vi "ABR3-Read Data.vi"(0 "Path":path, 11 "error in (no error)":errorcluster) -> (4 "Header":T3, 6 "Neural":dbl[][](array[numeric]), 8 "CM":dbl[][](array[numeric]), 10 "I-O":dbl[][](array[numeric]), 14 "Analysis":T1, 15 "error out":errorcluster)   [LabVIEW 2020]
uses:
  TypeDefs/ABR3-Analysis State.ctl
  Threshold Estimation VIs/ABR3-Threshold Estimation Result.ctl
  epl-vi-lib/Utility VIs/Array Manipulation VIs/Irregular Array Subset (DBL).vi
  epl-vi-lib/Utility VIs/Array Manipulation VIs/Array-Dimensions (2D).vi
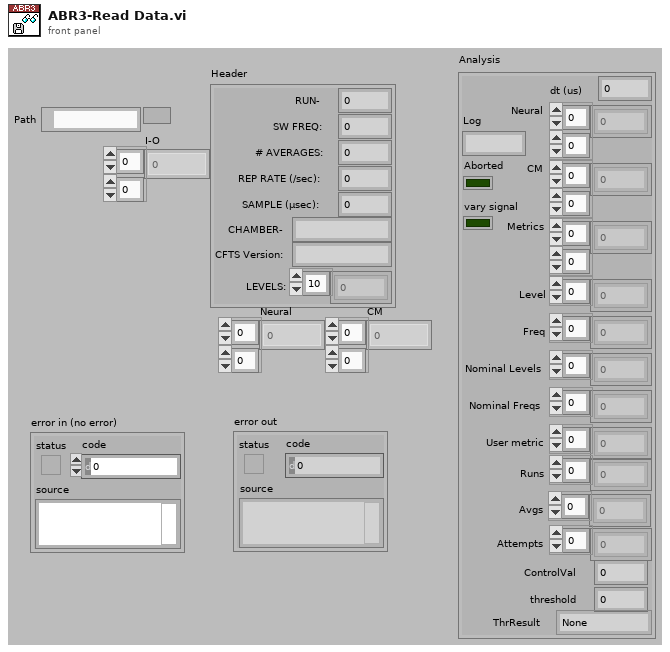
[diagram p1: front panel]
types:
  T1 = typedef "ABR3-Analysis State.ctl" = cluster{"dt (us)":dbl, "Neural":dbl[][], "CM":dbl[][], "Metrics":dbl[][], "Level":dbl[], "Freq":dbl[], "Nominal Levels":dbl[], "Nominal Freqs":dbl[], "User metric":dbl[], "Runs":i32[], "Avgs":i32[], "Attempts":i32[], "Log":string, "Aborted":bool, "ControlVal":dbl, "threshold":dbl, "vary signal":bool, "ThrResult":T2}
  T2 = typedef "ABR3-Threshold Estimation Result.ctl" = enum16{"None", "Power", "Sigmoid", "Power (noisy)", "Suprathreshold", "Invalid"}
  T3 = cluster{"RUN-":i32, "SW FREQ:":dbl, "# AVERAGES:":i32, "REP RATE (/sec):":dbl, "SAMPLE (µsec):":dbl, "CHAMBER-":string, "CFTS Version: ":string, "LEVELS:":dbl[]}
  T4 = typedef "ABR-Data Header.ctl" = cluster{"RUN-":i32, "SW FREQ:":dbl, "# AVERAGES:":i32, "REP RATE (/sec):":dbl, "SAMPLE (µsec):":dbl, "CHAMBER-":string, "CFTS Version: ":string, "LEVELS:":dbl[], "Date":timestamp, "Threshold:":dbl}
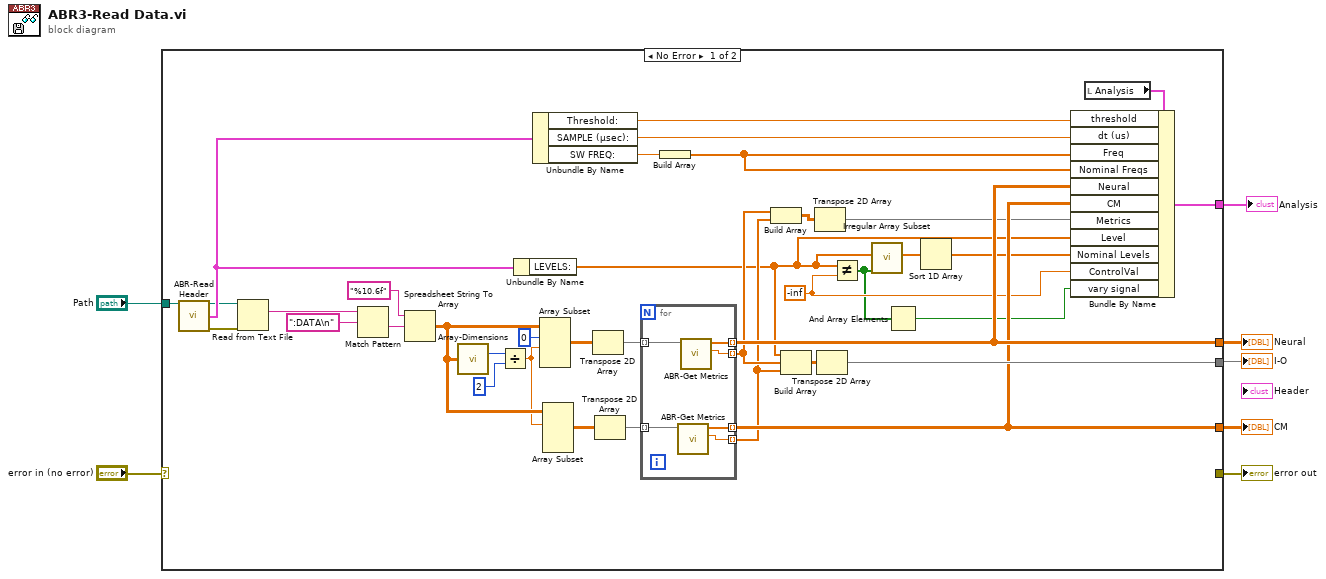
[diagram p0: block diagram]
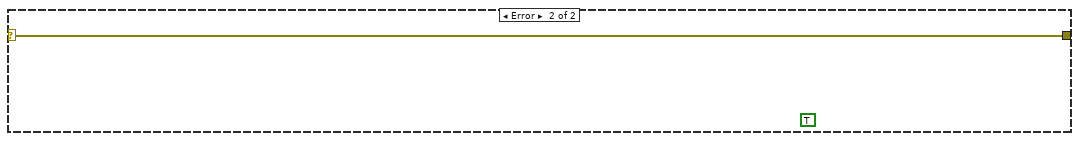
[diagram p2: hidden frame]
diagram:
  n1 = case shown="No Error" "error in (no error)" {
    selector: "error in (no error)" -> [_ w51]
    tunnel: [_ w51] -> w6
    tunnel: "Path" -> [w10 _]
    tunnel: [w41 _] -> w4
    tunnel: [w40 _] -> w3
    tunnel: [w43 _] -> w2
    tunnel: [w42 _] -> w1
    frame No Error {
      w18 = -inf
      n2 = call "ABR-Read Header.vi"("Path"=w10) -> ("Path (thru)"=w11:path, "Header"=w12:T4, "error out"=w9:errorcluster)  [unwired: 12 in]
      n3 = Read from Text File(file (use dialog)=w11, error in=w9) -> (text=w44:string)  [unwired: 2 in, 3 out]
      n4 = Match Pattern(string=w44, regular expression=":DATA\n" ("search string/char (-)")) -> (after substring=w31:string)  [unwired: 1 in, 3 out]
      n5 = Spreadsheet String To Array(format string="%10.6f" ("spreadsheet string"), spreadsheet string=w31) -> (array=w34:dbl[][])  [unwired: 2 in]
      n6 = call-poly "Array-Dimensions.vi"("2D Array"=w34) -> ("# rows"=w38:i32)  [unwired: 13 in, 1 out]
      n7 = Divide(x=w38, y=2) -> (x/y=w32:dbl)
      n8 = Unbundle By Name(w12) -> ("LEVELS:"=w17:dbl[])
      n9 = Unbundle By Name(w12) -> ("Threshold:"=w8:dbl, "SAMPLE (µsec):"=w25:dbl, "SW FREQ:"=w26:dbl)
      n10 = Array Subset(array=w34, index (row)=0 ("index"), length (row)=w32) -> (w35:dbl[][])  [unwired: 2 in]
      n11 = Array Subset(array=w34, index (row)=w32) -> (w33:dbl[][])  [unwired: 3 in]
      n12 = Transpose 2D Array(2D array=w35) -> (transposed array=w29:dbl[][])
      n13 = Transpose 2D Array(2D array=w33) -> (transposed array=w28:dbl[][])
      n14 = for {
        tunnel: w29 -> [w46] mode=indexing
        tunnel: w28 -> [w45] mode=indexing
        tunnel: [w50] -> w41 mode=indexing
        tunnel: [w49] -> w40 mode=indexing
        tunnel: [w48] -> w20 mode=indexing
        tunnel: [w47] -> w19 mode=indexing
        n15 = call "ABR-Get Metrics.vi"("Data in"=w45) -> ("spread value"=w47:dbl, "Data out"=w49:dbl[])  [unwired: 8 in, 1 out]
        n16 = call "ABR-Get Metrics.vi"("Data in"=w46) -> ("spread value"=w48:dbl, "Data out"=w50:dbl[])  [unwired: 8 in, 1 out]
      }
      n17 = Build Array(w26) -> (w24:dbl[])
      n18 = Build Array(w20, w19) -> (w22:dbl[][])
      n19 = Build Array(w17, w20, w19) -> (w27:dbl[][])
      n20 = Transpose 2D Array(2D array=w22) -> (transposed array=w21:dbl[][])
      n21 = Transpose 2D Array(2D array=w27) -> (transposed array=w43:dbl[][])
      n22 = Not Equal?(x=w17, y=w18) -> (x != y?=w14:bool[])
      n23 = call-poly "Irregular Array Subset.vi"("Mask"=w14, "Array"=w17) -> ("Array Subset"=w16:dbl[])  [unwired: 8 in, 1 out]
      n24 = And Array Elements(Boolean array=w14) -> (logical AND=w13:bool)
      n25 = Sort 1D Array(array=w16) -> (sorted array=w15:dbl[])
      n26 = local read "Analysis"() -> (w23:T1)
      n27 = Bundle By Name(cluster=w23, "threshold"=w8, "dt (us)"=w25, "Freq"=w24, "Nominal Freqs"=w24, "Neural"=w41, "CM"=w40, "Metrics"=w21, "Level"=w17, "Nominal Levels"=w15, "ControlVal"=w18, "vary signal"=w13) -> (w42:T1)
    }
    frame Error {
      (unwired) TRUE ("cancelled")
    }
  }
  "error out" <- w6
  "Neural" <- w4
  "CM" <- w3
  "I-O" <- w2
  "Analysis" <- w1
